vi "5-5Daqmx.vi"() -> ()   [LabVIEW 2024]
uses:
  <vilib>/DAQmx/read.llb/DAQmx Read (Analog 1D DBL NChan 1Samp).vi
  <vilib>/DAQmx/create/channels.llb/DAQmx Create Channel (AI-Temperature-Thermocouple).vi
  <vilib>/DAQmx/miscellaneous.llb/DAQmx Fill In Error Info.vi
  <vilib>/Utility/file.llb/Write Delimited Spreadsheet (string).vi
  <vilib>/Utility/file.llb/Write Delimited Spreadsheet (DBL).vi
  <resource>/objmgr/daqmx.rc
  <vilib>/DAQmx/read.llb/DAQmx Read (Analog DBL 1Chan 1Samp).vi
panel:
  in  "Stop Button 3":bool
  out "XY Graph":cluster{dbl[], dbl[]}[](graph)
  out "time domein baska yol":dbl[](array[numeric])
  out "time domein":dbl[](array[numeric])
  out "elapsed time":dbl
  in  "Stop Button 2":bool
  in  "seconds per data point 2":dbl
  in  "AI.ADCTimingMode 2":i32(ring)=16097 items=["Automatic"=16097, "High Resolution"=10195, "High Speed"=14712, "Best 50 Hz Rejection"=14713, "Best 60 Hz Rejection"=14714, "Custom"=10137]
  in  "thermocouple type 2":i32(ring)=10072 items=["J"=10072, "K"=10073, "N"=10077, "R"=10082, "S"=10085, "T"=10086, "B"=10047, "E"=10055]
  in  "physical channels 2":tag
  in  "seconds per data point":dbl
  in  "Stop Button":bool
  in  "AI.ADCTimingMode":i32(ring)=16097 items=["Automatic"=16097, "High Resolution"=10195, "High Speed"=14712, "Best 50 Hz Rejection"=14713, "Best 60 Hz Rejection"=14714, "Custom"=10137]
  out "Waveform Chart":dbl(graph)
  out "temperature":dbl format="%0.2f"
  in  "thermocouple type":i32(ring)=10072 items=["J"=10072, "K"=10073, "N"=10077, "R"=10082, "S"=10085, "T"=10086, "B"=10047, "E"=10055]
  in  "physical channels":tag
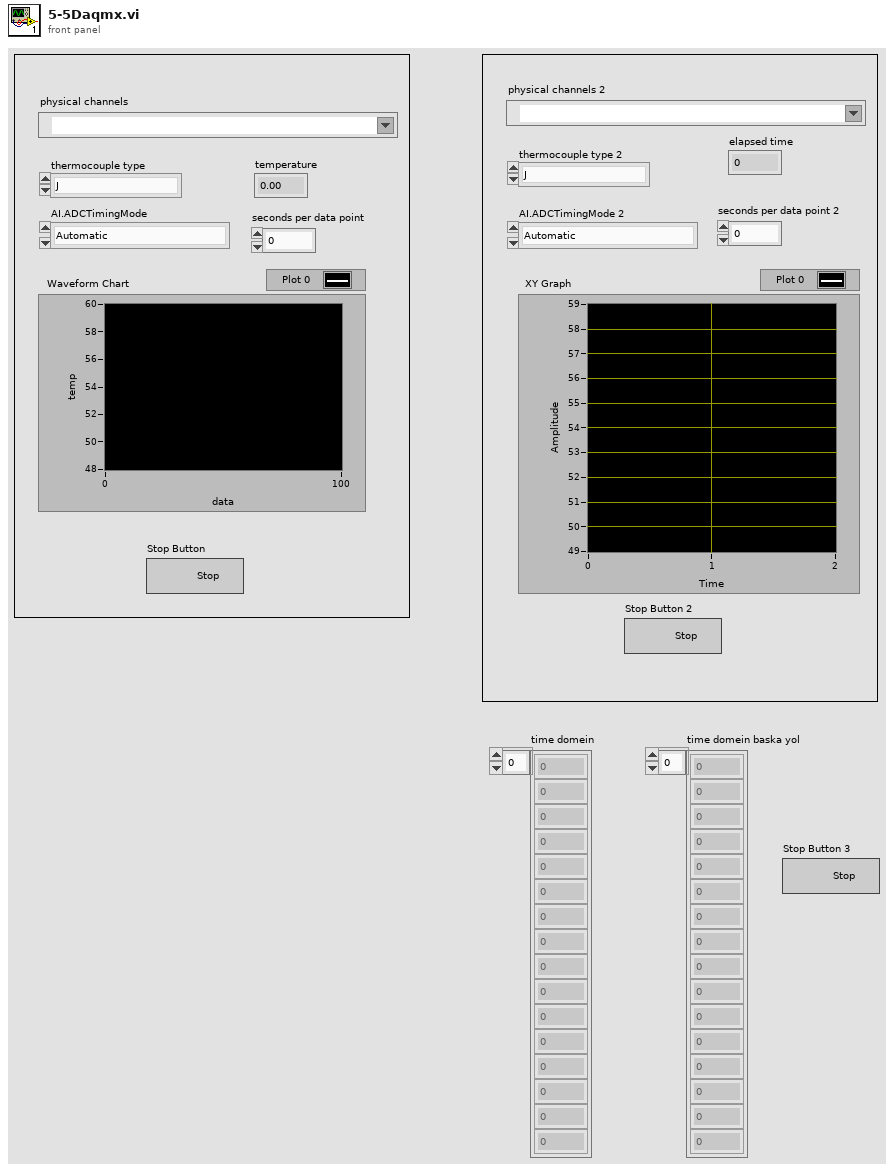
[diagram p1: front panel]
types:
  T1 = enum16{"open", "replace", "create", "open or create", "replace or create", "replace or create with confirmation"}
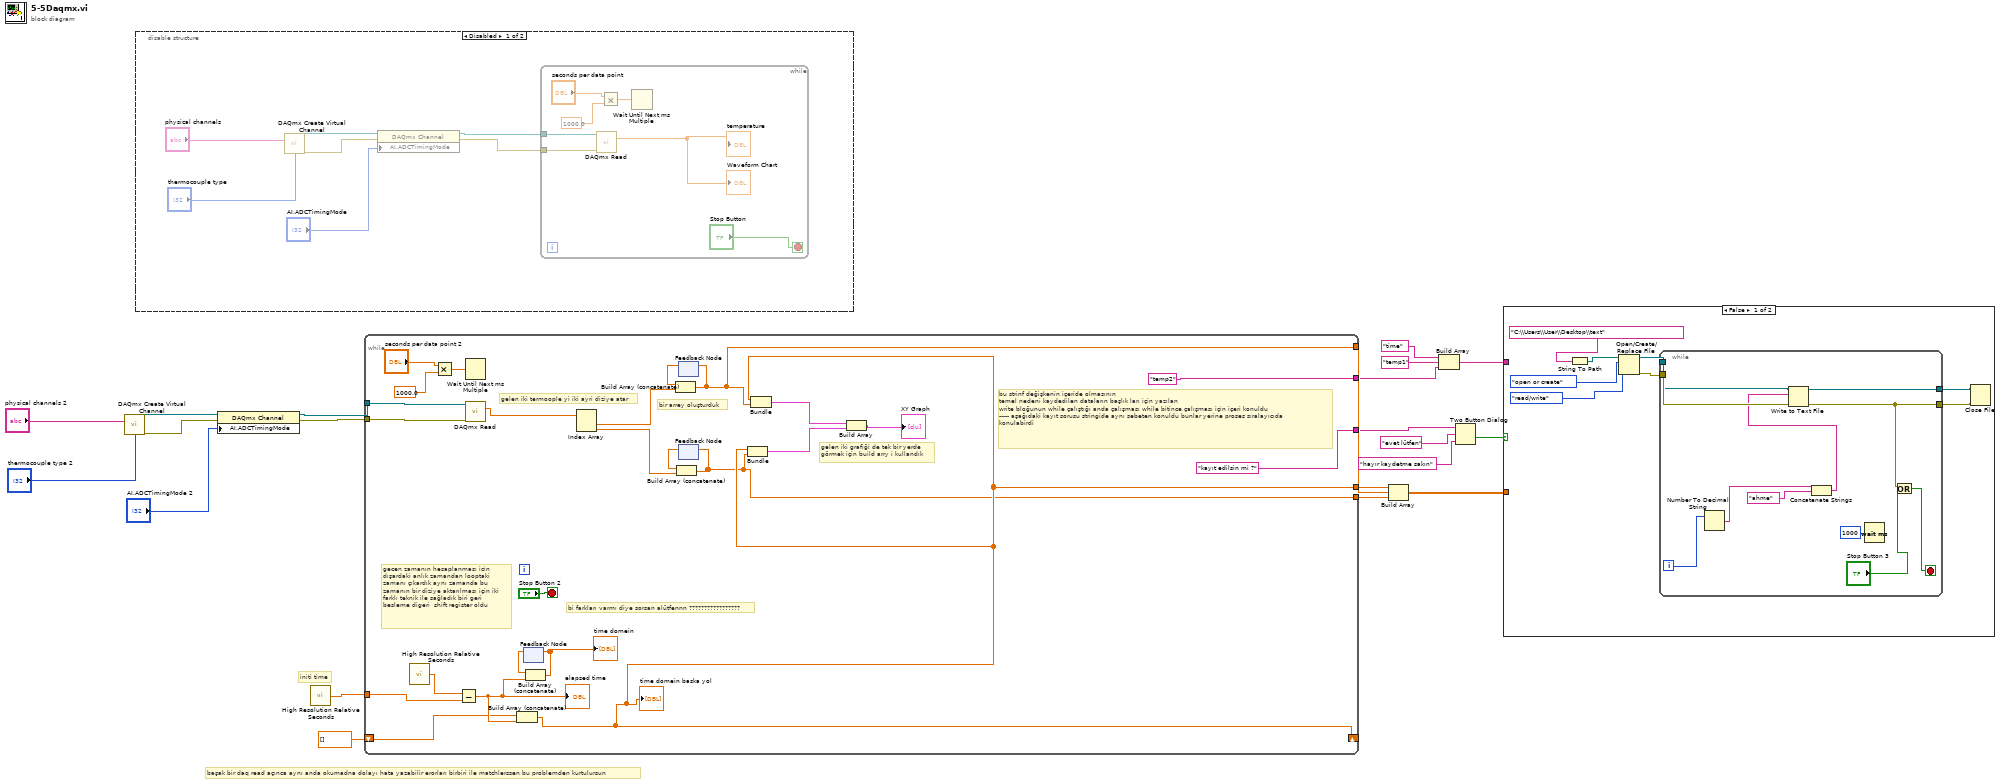
[diagram p0: block diagram]
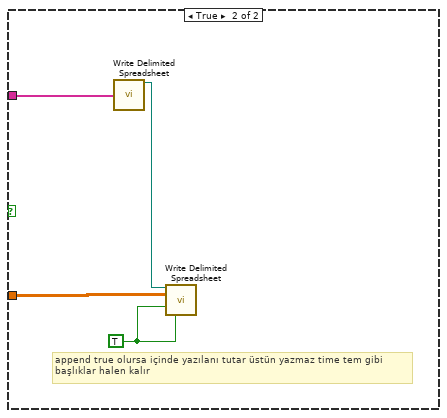
[diagram p2: hidden frame]
diagram:
  # "başak bir daq read açınca aynı anda okumadna dolayı hata yazabilir erorları birbiri ile matchlerssen bu problemden kurtulursun"
  # "initi time"
  n1 = call-poly <vilib>:"DAQmx Create Virtual Channel.vi"("physical channels"="physical channels 2", "thermocouple type"="thermocouple type 2") -> ("task out"=w18:refnum<k21>, "error out"=w17:errorcluster)  [unwired: 12 in]
  n2 = disable-structure shown="Disabled" {
    frame Disabled {
      n3 = call-poly <vilib>:"DAQmx Create Virtual Channel.vi"("physical channels"="physical channels", "thermocouple type"="thermocouple type") -> ("task out"=w25:refnum<k21>, "error out"=w24:errorcluster)  [unwired: 12 in]
      n4 = property class="DAQmx Channel"(reference=w25, error in=w24, "AI.ADCTimingMode"="AI.ADCTimingMode") -> (reference out=w22:refnum<k21>, error out=w23:errorcluster)
      n5 = while {
        tunnel: w23 -> [w34]
        tunnel: w22 -> [w33]
        stop <- "Stop Button" stop-if-true
        n6 = call-poly <vilib>:"DAQmx Read.vi"("task/channels in"=w33, "error in"=w34) -> ("data"=→"temperature" →"Waveform Chart":dbl)  [unwired: 11 in, 2 out]
        n7 = Multiply(x="seconds per data point", y=1000.0) -> (x*y=w31:dbl)
        n8 = Wait Until Next ms Multiple(millisecond multiple=w31) -> ()  [unwired: 1 out]
      }
    }
    frame Enabled {
    }
  }
  n9 = property class="DAQmx Channel"(reference=w18, error in=w17, "AI.ADCTimingMode"="AI.ADCTimingMode 2") -> (reference out=w15:refnum<k21>, error out=w16:errorcluster)
  n10 = call <vilib>:"High Resolution Relative Seconds.vi"() -> ("relative seconds"=w14:dbl)
  n11 = while {
    tunnel: w16 -> [w56]
    tunnel: w15 -> [w55]
    tunnel: w14 -> [w53]
    shift-right: [w40] -> _
    shift-left: dbl[] [] -> [w50]
    tunnel: [w40] -> w12
    tunnel: [w39] -> w11
    tunnel: [w38] -> w10
    tunnel: ["temp2"] -> w5
    tunnel: ["kayıt edilsin mi ?" ("message")] -> w1
    stop <- "Stop Button 2" stop-if-true
    # "bu strinf değişkenin içeride olmasının \ntemel nedeni kaydedilen dataların başlık ları için yazılan \nwrite bloğunun while çalıştığı anda çalışması while bitince çalışması için içeri konuldu \n----- aşağıdaki kayıt sorusu stringide aynı sebeten konuldu bunlar yerine proses sıralayıcıda \nkonulabirdi"
    # "gelen iki grafiği de tek bir yerde \ngörmek için build arry i kullandık"
    # "bir arrey oluşturduk"
    # "bi farkları varmı diye sorsan alütfennn ?????????????????"
    # "gelen iki termoople yi iki ayri diziye atar"
    # "gecen zamanın hesaplanması icin dışardaki anlık zamandan looptaki zamanı çıkardık aynı zamanda bu zamanın bir diziye aktarılması için iki farklı teknik ile sağladık biri geri besleme digeri  shift register oldu"
    n12 = call <vilib>:"High Resolution Relative Seconds.vi"() -> ("relative seconds"=w54:dbl)
    n13 = Multiply(x="seconds per data point 2", y=1000.0) -> (x*y=w59:dbl)
    n14 = Subtract(x=w54, y=w53) -> (x-y=w51:dbl)
    "elapsed time" <- w51
    n15 = Wait Until Next ms Multiple(millisecond multiple=w59) -> ()  [unwired: 1 out]
    n16 = call-poly <vilib>:"DAQmx Read.vi"("task/channels in"=w55, "error in"=w56) -> ("data"=w49:dbl[])  [unwired: 11 in, 2 out]
    n17 = Build Array (concatenate)(w50, w51) -> (w40:dbl[])
    "time domein baska yol" <- w40
    n18 = feedback #1() -> (w52:dbl[])  [unwired: 1 in]
    n19 = Build Array (concatenate)(w52, w51) -> (w41:dbl[])
    "time domein" <- w41
    n20 = feedback-in #1(w41) -> ()
    n21 = Index Array(array=w49) -> (element #1=w46:dbl, element #2=w47:dbl)  [unwired: 2 in]
    n22 = feedback #2() -> (w45:dbl[])  [unwired: 1 in]
    n23 = Build Array (concatenate)(w45, w46) -> (w38:dbl[])
    n24 = feedback-in #2(w38) -> ()
    n25 = feedback #3() -> (w48:dbl[])  [unwired: 1 in]
    n26 = Build Array (concatenate)(w48, w47) -> (w39:dbl[])
    n27 = feedback-in #3(w39) -> ()
    n28 = Bundle(w40, w39) -> (w44:cluster{dbl[], dbl[]})  [unwired: 1 in]
    n29 = Bundle(w40, w38) -> (w43:cluster{dbl[], dbl[]})  [unwired: 1 in]
    n30 = Build Array(w43, w44) -> (→"XY Graph":cluster{dbl[], dbl[]}[])
  }
  n31 = Build Array(w12, w10, w11) -> (w9:dbl[][])
  n32 = Build Array("time", "temp1", w5) -> (w6:string[])
  n33 = Two Button Dialog(message=w1, 1:"hayır kaydetme sakın" ("F button name (\"Cancel\")"), 2:"evet lütfen" ("T button name (\"OK\")")) -> (T button?=w4:bool)
  n34 = case shown="False" w4 {
    tunnel: w9 -> [_ w83]
    tunnel: w6 -> [_ w82]
    frame False {
      n35 = String To Path(string="C:\\Users\\User\\Desktop\\text") -> (path=w67:path)
      n36 = Open/Create/Replace File(file path (use dialog)=w67, operation (0:open)=T1."open or create", access (0:read/write)=enum16{"read/write", "read-only", "write-only"}."read/write") -> (refnum out=w63:refnum<file>, error out=w64:errorcluster)  [unwired: 3 in, 1 out]
      n37 = while {
        tunnel: w64 -> [w79]
        tunnel: w63 -> [w78]
        tunnel: [w76] -> w62
        tunnel: [w71] -> w61
        i -> [w75]
        stop <- w69 stop-if-true
        n38 = Number To Decimal String(number=w75) -> (decimal integer string=w74:string)  [unwired: 1 in]
        n39 = Concatenate Strings(w74, "ahme") -> (w72:string)
        n40 = Write to Text File(file (use dialog)=w78, text=w72, error in=w79) -> (refnum out=w76:refnum<file>, error out=w71:errorcluster)  [unwired: 1 in, 1 out]
        n41 = Wait (ms)(milliseconds to wait=u32 1000) -> ()  [unwired: 1 out]
        n42 = Or(x=w71, y="Stop Button 3") -> (x .or. y?=w69:bool)
      }
      n43 = Close File(refnum=w62, error in=w61) -> ()  [unwired: 2 out]
    }
    frame True {
      w80 = TRUE ("transpose? (no:F)")
      # "append true olursa içinde yazılanı tutar üstün yazmaz time tem gibi \nbaşlıklar halen kalır"
      n44 = call-poly <vilib>:"Write Delimited Spreadsheet.vi"("1D data"=w82) -> ("new file path (Not A Path if cancelled)"=w81:path)  [unwired: 13 in, 1 out]
      n45 = call-poly <vilib>:"Write Delimited Spreadsheet.vi"("file path (dialog if empty)"=w81, "2D data"=w83, "append to file? (new file:F)"=w80, "transpose? (no:F)"=w80) -> ()  [unwired: 10 in, 2 out]
    }
  }
